vi "Laser_Ratio.vi"(2 "Numeric 3":i16, 3 "Laser 470 nm (blue)":dbl) -> (0 "Numeric":u16, 1 "Numeric 2":u16)   [LabVIEW 2009]
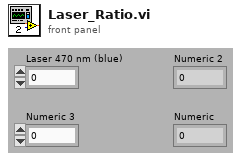
[diagram p1: front panel]
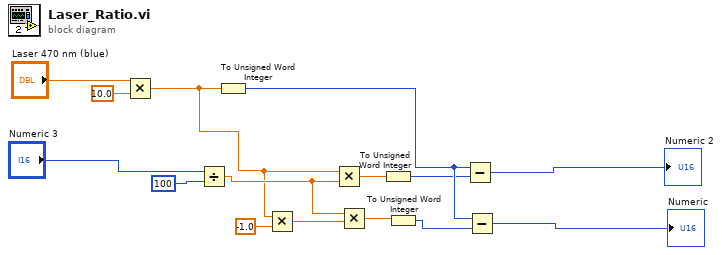
[diagram p0: block diagram]
diagram:
  n1 = Multiply(x="Laser 470 nm (blue)", y=10.0) -> (x*y=w2:dbl)
  n2 = Divide(x="Numeric 3", y=i16 100) -> (x/y=w15:dbl)
  n3 = To Unsigned Word Integer(number=w2) -> (unsigned 16bit integer=w10:u16)
  n4 = Multiply(x=w2, y=-1.0) -> (x*y=w13:dbl)
  n5 = Multiply(x=w2, y=w15) -> (x*y=w6:dbl)
  n6 = Multiply(x=w15, y=w13) -> (x*y=w14:dbl)
  n7 = To Unsigned Word Integer(number=w6) -> (unsigned 16bit integer=w7:u16)
  n8 = To Unsigned Word Integer(number=w14) -> (unsigned 16bit integer=w11:u16)
  n9 = Subtract(x=w10, y=w7) -> (x-y=→"Numeric 2":u16)
  n10 = Subtract(x=w10, y=w11) -> (x-y=→"Numeric":u16)
